vi "Read Write Background Image (SubVI).vi"(5 "Image Width":u16, 7 "Image Height":u16) -> ()   [LabVIEW 2015]
uses:
  <vilib>/rvi/DataTransferAndStorage/Container/XNode/niFpgaContainer.xnode
  <vilib>/rvi/Memory/Memory_Emulation/niFpgaMemoryEmulationDramWriteAndRequestData.vi
  <vilib>/rvi/Memory/Memory_Emulation/niFpgaMemoryFastEmulationDramWriteAndRequestData.vi
  <vilib>/rvi/FIFO/Fifo_Resource/nirvififoEmulationWrite.vi
  Common/Controls (FPGA)/Receive BG Image.ctl
  <vilib>/rvi/interface/RandomDataEmulation/nirviRandomDataFpgaMultiElementTemplate.vi
  <vilib>/rvi/FIFO/Fifo_Resource/nirvififoEmulationRead.vi
  <vilib>/rvi/Memory/Memory_Emulation/niFpgaMemoryEmulationDramRetrieveData.vi
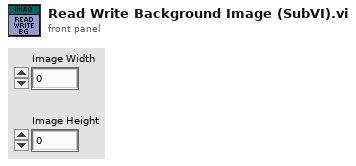
[diagram p1: front panel]
types:
  T1 = typedef "Receive BG Image.ctl" = enum16{"Packet 1", "Packet 2"}
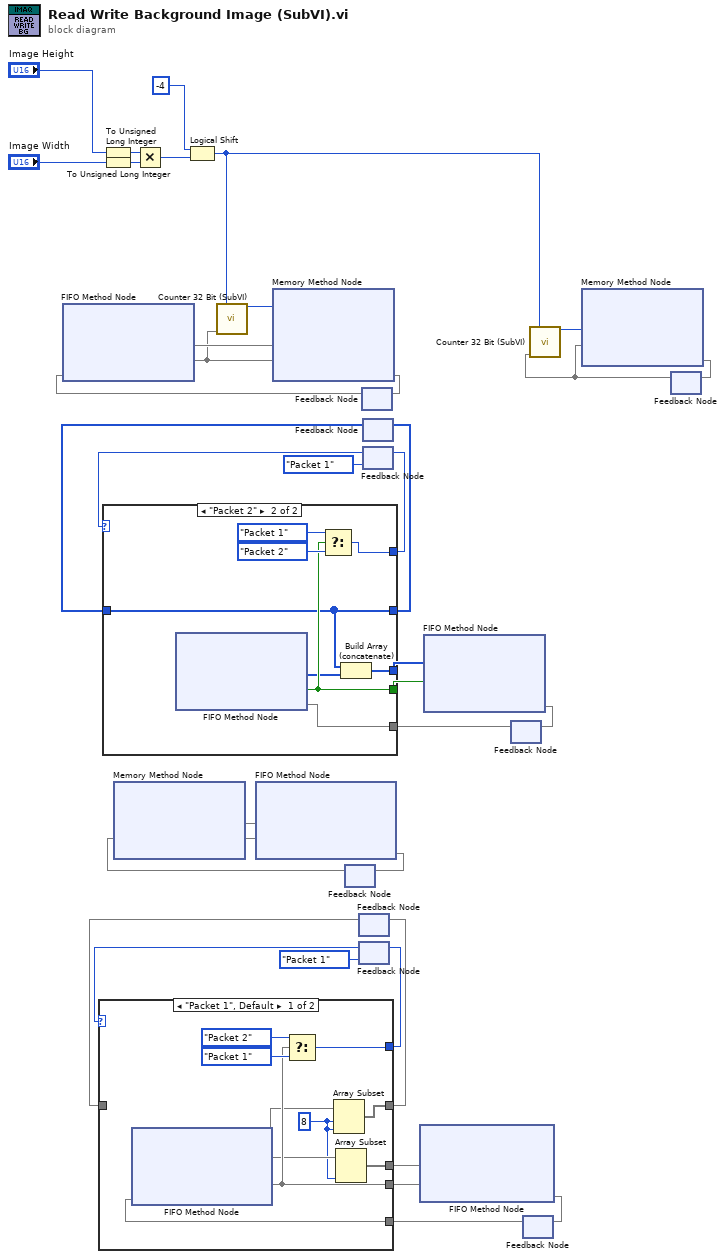
[diagram p0: block diagram]
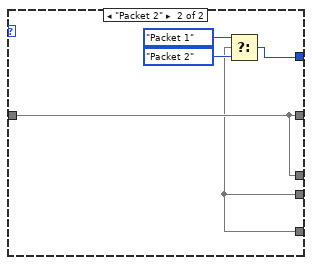
[diagram p2: hidden frame]
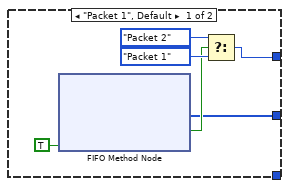
[diagram p3: hidden frame]
diagram:
  n1 = To Unsigned Long Integer(number="Image Height") -> (unsigned 32bit integer=w35:u32)
  n2 = To Unsigned Long Integer(number="Image Width") -> (unsigned 32bit integer=w36:u32)
  n3 = Multiply(x=w35, y=w36) -> (x*y=w33:u32)
  n4 = Logical Shift(y=i16 -4, x=w33) -> (x << y=w37:u32)
  n5 = feedback #1() -> (w19)  [unwired: 1 in]
  n6 = xnode ("Memory Method Node")("Ready for Output"=w19) -> ("Data"=w18, "Output Valid"=w21)  [unwired: 1 in, 1 out]
  n7 = xnode ("FIFO Method Node")("Element"=w18, "Input Valid"=w21) -> ("Ready for Input"=w20)  [unwired: 1 in, 1 out]
  n8 = feedback-in #1(w20) -> ()
  n9 = feedback #2() -> (w24)  [unwired: 1 in]
  n10 = feedback #3(Receive_BG_Image."Packet 1") -> (w27:T1)
  n11 = feedback #4() -> (w3)  [unwired: 1 in]
  n12 = xnode ("FIFO Method Node")("Ready for Output"=w3) -> ("Element"=w4, "Output Valid"=w2)  [unwired: 1 in, 1 out]
  n13 = call "Counter 32 Bit (SubVI).vi"("Max. Count"=w37, "Enable"=w2) -> ("Count"=w1:u32)  [unwired: 11 in, 2 out]
  n14 = xnode ("Memory Method Node")("Address"=w1, "Data"=w4, "Input Valid"=w2) -> ("Ready for Input"=w14)  [unwired: 1 in, 1 out]
  n15 = feedback-in #4(w14) -> ()
  n16 = feedback #5() -> (w7:u8[])  [unwired: 1 in]
  n17 = feedback #6(Receive_BG_Image."Packet 1") -> (w10:T1)
  n18 = feedback #7() -> (w6)  [unwired: 1 in]
  n19 = case shown="\"Packet 2\"" w10 {
    tunnel: [_ w48] -> w13
    tunnel: [w42 w50] -> w11
    tunnel: [w40 w46] -> w8
    tunnel: w7 -> [_ w46]
    tunnel: w6 -> [_ w47]
    tunnel: [_ w44] -> w5
    frame "Packet 1", Default {
      n20 = xnode ("FIFO Method Node")("Ready for Output"=TRUE) -> ("Element"=w40:u8[], "Output Valid"=w41:bool)  [unwired: 1 in, 1 out]
      n21 = Select(t=Receive_BG_Image."Packet 2", s=w41, f=Receive_BG_Image."Packet 1") -> (s? t:f=w42:T1)
    }
    frame "Packet 2" {
      n22 = xnode ("FIFO Method Node")("Ready for Output"=w47) -> ("Element"=w45:u8[], "Output Valid"=w48:bool)  [unwired: 1 in, 1 out]
      n23 = Select(t=Receive_BG_Image."Packet 1", s=w48, f=Receive_BG_Image."Packet 2") -> (s? t:f=w50:T1)
      n24 = Build Array (concatenate)(w46, w45) -> (w44:u8[])
    }
  }
  n25 = feedback-in #5(w8) -> ()
  n26 = feedback-in #6(w11) -> ()
  n27 = xnode ("FIFO Method Node")("Element"=w5, "Input Valid"=w13) -> ("Ready for Input"=w12)  [unwired: 1 in, 1 out]
  n28 = feedback-in #7(w12) -> ()
  n29 = feedback #8() -> (w23)  [unwired: 1 in]
  n30 = case shown="\"Packet 1\", Default" w27 {
    tunnel: [w56 w61] -> w30
    tunnel: [w59 w64] -> w28
    tunnel: [w53 w62] -> w25
    tunnel: w24 -> [_ w62]
    tunnel: w23 -> [w57 w61]
    tunnel: [w55 w62] -> w22
    frame "Packet 1", Default {
      w52 = 8 ("length")
      n31 = xnode ("FIFO Method Node")("Ready for Output"=w57) -> ("Element"=w54, "Output Valid"=w56)  [unwired: 1 in, 1 out]
      n32 = Select(t=Receive_BG_Image."Packet 2", s=w56, f=Receive_BG_Image."Packet 1") -> (s? t:f=w59:T1)
      n33 = Array Subset(array=w54, index=w52, length=w52) -> (w53:void[])
      n34 = Array Subset(array=w54, length=w52) -> (w55:void[])  [unwired: 1 in]
    }
    frame "Packet 2" {
      n35 = Select(t=Receive_BG_Image."Packet 1", s=w61, f=Receive_BG_Image."Packet 2") -> (s? t:f=w64:T1)
    }
  }
  n36 = feedback-in #2(w25) -> ()
  n37 = feedback-in #3(w28) -> ()
  n38 = xnode ("FIFO Method Node")("Element"=w22, "Input Valid"=w30) -> ("Ready for Input"=w29)  [unwired: 1 in, 1 out]
  n39 = feedback-in #8(w29) -> ()
  n40 = feedback #9() -> (w17)  [unwired: 1 in]
  n41 = call "Counter 32 Bit (SubVI).vi"("Max. Count"=w37, "Enable"=w17) -> ("Count"=w16:u32)  [unwired: 11 in, 2 out]
  n42 = xnode ("Memory Method Node")("Address"=w16, "Input Valid"=w17) -> ("Ready for Input"=w15)  [unwired: 1 in, 1 out]
  n43 = feedback-in #9(w15) -> ()
